vi "Close Connection.vi"(8 "error in":errorcluster, 11 "TCP slave in":refnum<class "TCP Server.lvclass">) -> (0 "error out":errorcluster)   [LabVIEW 2021, in "WebSockets.lvlib" / "TCP Server.lvclass"]
doc: "Closes the TCP connection stored in the class."
uses:
  TCP Server.lvclass
  D:/my_projects/projects/Algorithms/Labview/21/WebSockets/WebSockets/WebSocket/WebSocket.lvclass
  WebSocket/WebSocket.lvclass/WebSocket.ctl
  Sockets/Socket/Socket.lvclass
  TCP Server.lvclass/TCP Server.ctl
  WebSocket/WebSocket.lvclass
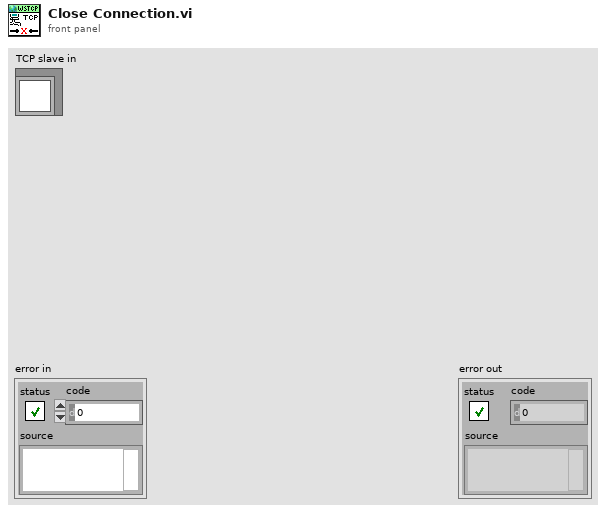
[diagram p1: front panel]
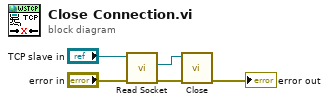
[diagram p0: block diagram]
diagram:
  n1 = call "Read Socket.vi"("error in (no error)"="error in", "WebSocket in"="TCP slave in") -> ("error out"=w2:errorcluster, "Socket"=w5:refnum<class "Socket.lvclass">)  [unwired: 7 in, 1 out]
  n2 = call-dynamic "Close.vi"("error in (no error)"=w2, "Socket in"=w5) -> ("error out"=→"error out":errorcluster)  [unwired: 9 in]
